vi "Display Measurement.vi"(8 "error in (no error)":errorcluster, 10 "Displayed Measurement (0: Voltage)":u16(ring) items=["Voltage", "Current", "Resistance"], 11 "VISA resource name":refnum<visa-resource-name>) -> (0 "error out":errorcluster, 3 "VISA resource name out":refnum<visa-resource-name>)   [LabVIEW 2017, in "Keithley 24XX.lvlib"]
doc: "Makes the display show the desired measurement.\n\n<B>Note:</B> This VI has absolutely no effect on the measurements taken, just which one is displayed on the front panel."
uses:
  <instrlib>/Keithley 24XX/Keithley 24XX.lvlib
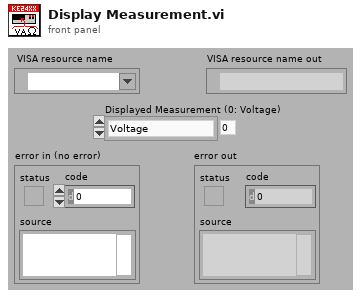
[diagram p1: front panel]
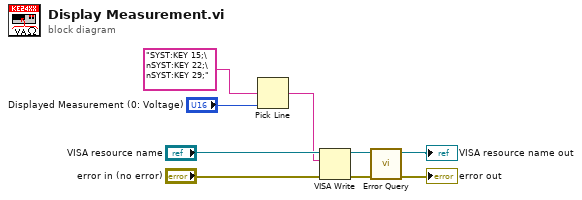
[diagram p0: block diagram]
diagram:
  n1 = Pick Line(multi-line string="SYST:KEY 15;\nSYST:KEY 22;\nSYST:KEY 29;", line index="Displayed Measurement (0: Voltage)") -> (output string=w5:string)  [unwired: 1 in]
  n2 = VISA Write(VISA resource name="VISA resource name", write buffer=w5, error in (no error)="error in (no error)") -> (VISA resource name out=w4:refnum<visa-resource-name>, error out=w1:errorcluster)  [unwired: 1 out]
  n3 = call <instrlib>:"Error Query.vi"("error in (no error)"=w1, "VISA resource name"=w4) -> ("error out"=→"error out":errorcluster, "VISA resource name out"=→"VISA resource name out":refnum<visa-resource-name>)  [unwired: 6 in, 2 out]
